vi "Pressure Sensor Test.vi"(0 "GEA2 Reference In":refnum<k24>, 11 "Error In":errorcluster) -> (4 "GEA2 Reference Out":refnum<k24>, 6 "Pass/Fail?":bool, 8 "Report Text":string, 15 "Error Out":errorcluster)   [LabVIEW 2016]
doc: "This VI performs the LED test. It first Writes the LED ERD to turn on all of the LEDs. Then prompts the user as to whether all LEDs are lit or not, for he Pass/Fail status."
uses:
  C:/Automation/DLLs/PC Dot Net/GeaCommunication.dll
  Common/LabVIEW GEA2 Toolkit/LabVIEW_GEA2_Toolkit.lvlibp/type defs/Source_Destination.ctl
  Common/LabVIEW GEA2 Toolkit/LabVIEW_GEA2_Toolkit.lvlibp/type defs/ERD Read Data In.ctl
  Common/LabVIEW GEA2 Toolkit/LabVIEW_GEA2_Toolkit.lvlibp/type defs/Data Type.ctl
  Common/LabVIEW GEA2 Toolkit/LabVIEW_GEA2_Toolkit.lvlibp
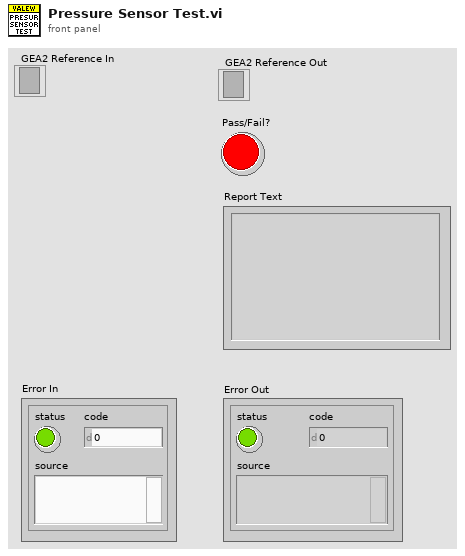
[diagram p1: front panel]
types:
  T1 = typedef "LabVIEW_GEA2_Toolkit.lvlibp/ERD Read Data In.ctl" = cluster{"ERD Number":u16, "Data Type":T2}
  T2 = typedef "LabVIEW_GEA2_Toolkit.lvlibp/Data Type.ctl" = enum16{"string", "boolean", "uint8_t", "uint16_t", "uint32_t", "uint64_t", "int8_t", "int16_t", "int32_t", "int64_t"}
  T3 = typedef "LabVIEW_GEA2_Toolkit.lvlibp/Source_Destination.ctl" = cluster{"Source":u8, "Destination":u8}
  T4 = typedef "LabVIEW_GEA2_Toolkit.lvlibp/ERD Read Data Out.ctl" = cluster{"ERD Number":u16, "Data":string}
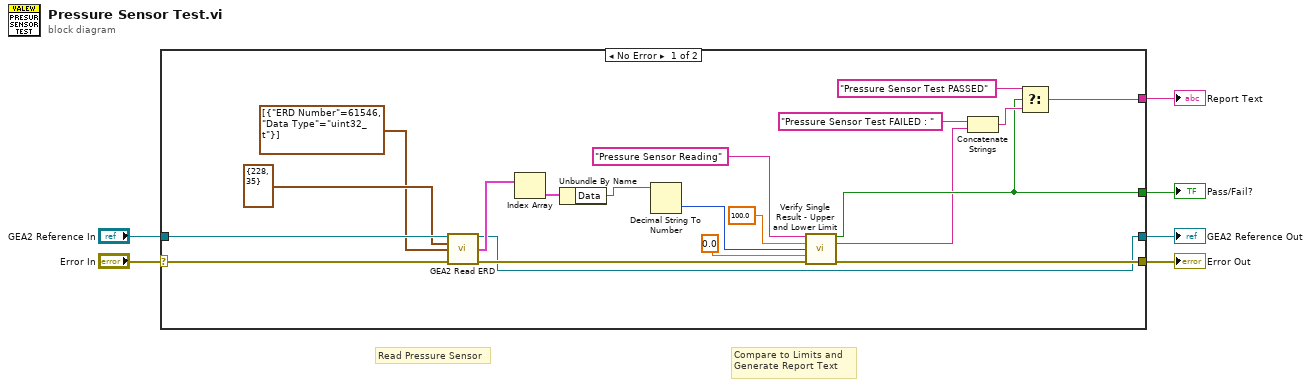
[diagram p0: block diagram]
diagram:
  # "Compare to Limits and\nGenerate Report Text"
  # "Read Pressure Sensor"
  n1 = case shown="No Error" "Error In" {
    selector: "Error In" -> [w24 w28]
    tunnel: "GEA2 Reference In" -> [w26 w27]
    tunnel: [w21 w28] -> w5
    tunnel: [w9 _] -> w4
    tunnel: [w13 w27] -> w3
    tunnel: [w7 _] -> w1
    frame No Error {
      n2 = call "GEA2 Read ERD.vi"("GEA2 Reference In"=w26, "GEA Inputs"=T3 {"Source"=228, "Destination"=35}, "Read ERD List"=T1[] [{"ERD Number"=61546, "Data Type"=enum."uint32_t"}], "Error In"=w24) -> ("GEA2 Reference Out"=w13:refnum<k24>, "ERD Data Out"=w20:T4[], "Error Out"=w22:errorcluster)  [unwired: 8 in, 1 out]
      n3 = Index Array(array=w20) -> (element=w19:T4)  [unwired: 1 in]
      n4 = Unbundle By Name(w19) -> ("Data"=w18:string)
      n5 = Decimal String To Number(string=w18) -> (number=w17:i32)  [unwired: 2 in, 1 out]
      n6 = call "Verify Single Result - Upper and Lower Limit.vi"("Name"="Pressure Sensor Reading", "Upper Limit"=100.0, "Value"=w17, "Lower Limit"=0.0, "Error In"=w22) -> ("Pass/Fail?"=w9:bool, "Report Text"=w8:string, "Error Out"=w21:errorcluster)  [unwired: 8 in]
      n7 = Concatenate Strings("Pressure Sensor Test FAILED : ", w8) -> (w11:string)
      n8 = Select(t="Pressure Sensor Test PASSED", s=w9, f=w11) -> (s? t:f=w7:string)
    }
    frame Error {
    }
  }
  "Error Out" <- w5
  "Pass/Fail?" <- w4
  "Report Text" <- w1
  "GEA2 Reference Out" <- w3
